vi "Autogenerated adjust limbus.vi"(0 "Range (Threshold 1)":cluster{"Lower value":sgl, "Upper value":sgl}={"Lower value"=140.0, "Upper value"=255.0}, 7 "error in":errorcluster) -> (20 "Fitted Circle (Find Circular Edge 1)":T2 {"Average SNR (dB)" format="%.2f"; "Average Strength" format="%.2f"; "Roundness (Real-World)" format="%.2f"; "Radius (Real-World)" format="%.2f"; "Center (Real-World)"."Y" format="%.2f"; "Center (Real-World)"."X" format="%.2f"; "Radius (Pixels)" format="%.2f"; "Center (Pixels)"."Y" format="%.2f"; "Center (Pixels)"."X" format="%.2f"}, 27 "error out":errorcluster)   [LabVIEW 2014]
uses:
  <vilib>/vision/Measure.llb/Edge Options.ctl
  <vilib>/vision/Measure.llb/Edge Polarity.ctl
  <vilib>/vision/NI_Vision_Development_Module.lvlib
panel:
  out "Image Out":T1(plugin-control)
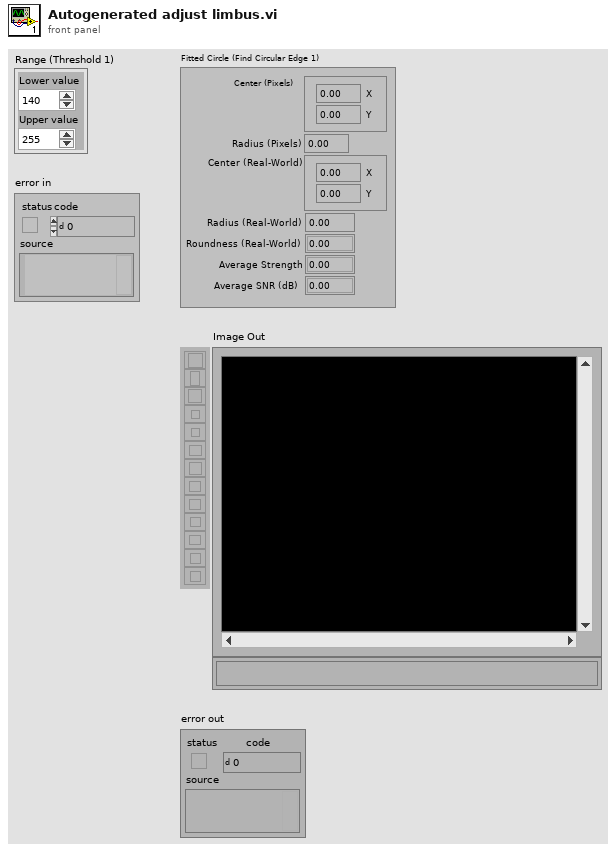
[diagram p1: front panel]
types:
  T1 = typedef "IMAQ Image.ctl" = refnum<image>
  T2 = cluster{"Center (Pixels)":cluster{"X":sgl, "Y":sgl}, "Radius (Pixels)":dbl, "Center (Real-World)":cluster{"X":sgl, "Y":sgl}, "Radius (Real-World)":dbl, "Roundness (Real-World)":dbl, "Average Strength":dbl, "Average SNR (dB)":dbl}
  T3 = typedef "Edge Options.ctl" = cluster{"Edge Polarity":T4, "Kernel Size":u32, "Width":u32, "Minimum Edge Strength":sgl, "Interpolation Type":enum32{"Zero Order", "Bilinear", "Quadratic", "Cubic", "Bilinear Fixed"}, "Data Processing Method":enum32{"Average", "Median"}}
  T4 = typedef "Edge Polarity.ctl" = u32
  T5 = cluster{"Search  Direction":u32, "Edge Options":T3, "Show Search Area":bool, "Show Search Lines":bool, "Show Edges Found":bool, "Show Result":bool, "Search Area Color":u32, "Search Lines Color":u32, "Edge Locations Color":u32, "Result Color":u32, "Overlay Group Name":string}
  T6 = cluster{"Process":enum16{"Get First Edge", "Get First + Last Edge", "Get All Edges", "Get Best Edge"}, "Step Size":i32, "Max Pixel Radius":i32}
  T7 = cluster{"Global Rectangle":i32[], "Contours":cluster{"ID":enum32{"External", "Internal"}, "Type":u32, "Coordinates":i32[]}[]}
  T8 = typedef "Image Type" = u32
  T9 = cluster{"histogram":u32[], "Minimal Value":sgl, "Maximal Value":sgl, "Starting Value":sgl, "Interval Width":sgl, "Mean Value":sgl, "Standard  Variation":sgl, "Area (pixels)":i32}
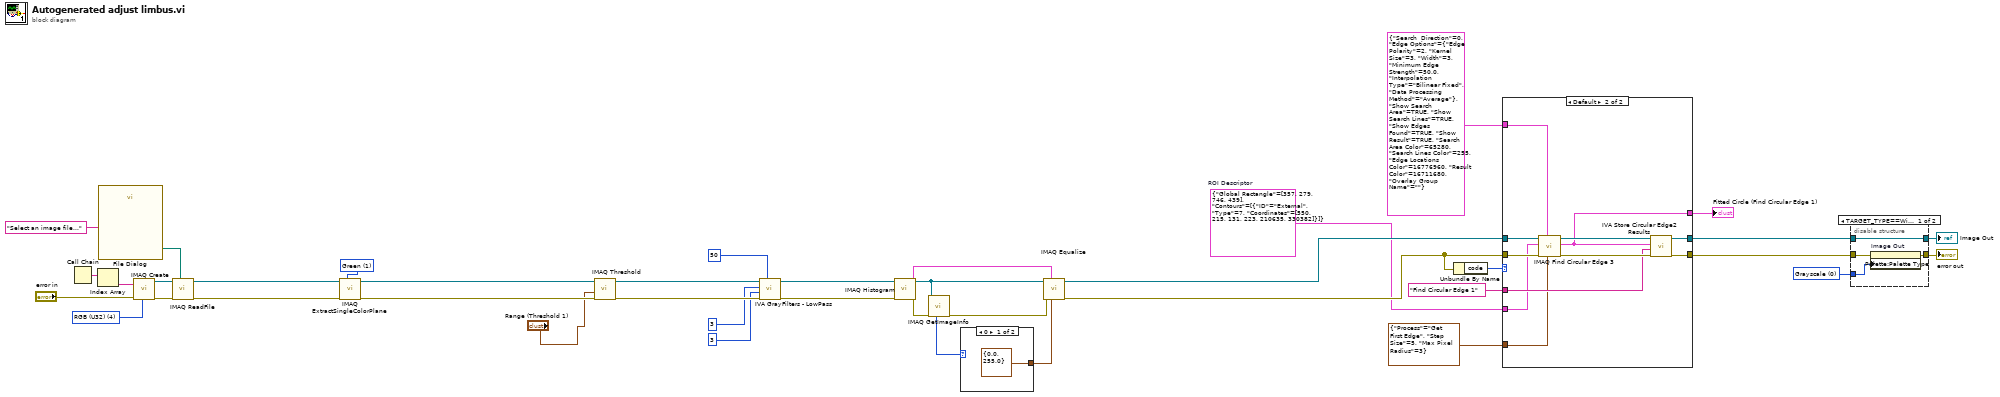
[diagram p0: block diagram]
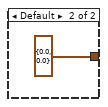
[diagram p4: hidden frame]
diagram:
  w1 = u32 0 items=["Grayscale", "Binary", "Gradient", "Rainbow", "Temperature", "User Defined"] ("Palette")
  w9 = T7 {"Global Rectangle"=[357, 279, 746, 439], "Contours"=[{"ID"=enum."External", "Type"=7, "Coordinates"=[550, 215, 131, 223, 210635, 330382]}]}  # ROI Descriptor
  w30 = 1 items=["Red", "Green", "Blue", "Hue", "Saturation", "Luminance", "Value", "Intensity"] ("Color Plane")
  w31 = T8 4 items=["Grayscale (U8)", "Grayscale (I16)", "Grayscale (SGL)", "Complex (CSG)", "RGB (U32)", "HSL (U32)", "RGB (U64)", "Grayscale (U16)"] ("Image Type")
  n1 = Call Chain() -> (call chain=w35:string[])
  n2 = Index Array(array=w35) -> (element=w34:string)  [unwired: 1 in]
  n3 = call "File Dialog"("prompt"="Select an image file...") -> ("selected path"=w32:path)  [unwired: 6 in, 8 out]
  n4 = call "IMAQ Create"("Image Name"=w34, "Image Type"=w31, "error in (no error)"="error in") -> ("New Image"=w38:T1, "error out"=w37:errorcluster)  [unwired: 1 in, 1 out]
  n5 = call "IMAQ ReadFile"("File Path"=w32, "error in (no error)"=w37, "Image"=w38) -> ("error out"=w39:errorcluster, "Image Out"=w29:T1)  [unwired: 2 in, 5 out]
  n6 = call "IMAQ ExtractSingleColorPlane"("Color Plane"=w30, "error in (no error)"=w39, "Image Src"=w29) -> ("error out"=w28:errorcluster, "Image Dst Out"=w26:T1)  [unwired: 1 in, 6 out]
  n7 = call "IMAQ Threshold"("error in (no error)"=w28, "Range"="Range (Threshold 1)", "Image Src"=w26) -> ("error out"=w25:errorcluster, "Image Dst Out"=w24:T1)  [unwired: 3 in, 4 out]
  n8 = call <vilib>:"IVA GrayFilters - LowPass.vi"("Tolerance"=50, "error in"=w25, "Filter size Y"=3, "Filter size X"=3, "Image In"=w24) -> ("error out"=w23:errorcluster, "Image Out"=w16:T1)  [unwired: 5 out]
  n9 = call "IMAQ Histogram"("error in (no error)"=w23, "Image"=w16) -> ("error out"=w15:errorcluster, "Histogram Report"=w18:T9)  [unwired: 3 in, 5 out]
  n10 = call "IMAQ GetImageInfo"("error in (no error)"=w15, "Image"=w16) -> ("error out"=w14:errorcluster, "Image Type"=w17:T8)  [unwired: 8 out]
  n11 = case shown="0" w17 {
    tunnel: [cluster{"Minimum":sgl, "Maximum":sgl} {"Minimum"=0.0, "Maximum"=255.0} ("Range") cluster{"Minimum":sgl, "Maximum":sgl} {"Minimum"=0.0, "Maximum"=0.0} ("Range")] -> w13
    frame 0 {
    }
    frame Default {
    }
  }
  n12 = call "IMAQ Equalize"("Range"=w13, "Histogram Report"=w18, "error in (no error)"=w14, "Image Src"=w16) -> ("error out"=w19:errorcluster, "Image Dst Out"=w12:T1)  [unwired: 2 in, 4 out]
  n13 = Unbundle By Name(w19) -> ("code"=w8:i32)
  n14 = case shown="Default" w8 {
    tunnel: T5 {"Search  Direction"=0, "Edge Options"={"Edge Polarity"=2, "Kernel Size"=3, "Width"=3, "Minimum Edge Strength"=50.0, "Interpolation Type"=enum."Bilinear Fixed", "Data Processing Method"=enum."Average"}, "Show Search Area"=TRUE, "Show Search Lines"=TRUE, "Show Edges Found"=TRUE, "Show Result"=TRUE, "Search Area Color"=65280, "Search Lines Color"=255, "Edge Locations Color"=16776960, "Result Color"=16711680, "Overlay Group Name"=""} ("Options") -> [_ w43]
    tunnel: w12 -> [w42 w53]
    tunnel: w19 -> [_ w52]
    tunnel: [_ w50] -> w11
    tunnel: [w42 w48] -> w3
    tunnel: "Find Circular Edge 1" ("Step Name") -> [_ w47]
    tunnel: w9 -> [_ w46]
    tunnel: T6 {"Process"=enum."Get First Edge", "Step Size"=5, "Max Pixel Radius"=3} ("Circle Fit Options") -> [_ w45]
    tunnel: [_ w44] -> w6
    frame -1074396199, -1074396198 {
      # "Discard Coordinate System Error"
    }
    frame Default {
      n15 = call "IMAQ Find Circular Edge 3"("Circle Fit Options"=w45, "Options"=w43, "error in (no error)"=w52, "ROI Descriptor"=w46, "Image"=w53) -> ("error out"=w51:errorcluster, "Fitted Circle"=w44:T2, "Image Out"=w49:T1)  [unwired: 2 in, 2 out]
      n16 = call <vilib>:"IVA Store Circular Edge2 Results.vi"("error in (no error)"=w51, "Step Name"=w47, "Fitted Circle"=w44, "Image in"=w49) -> ("error out"=w50:errorcluster, "Image dup"=w48:T1)  [unwired: 2 in, 4 out]
    }
  }
  "Fitted Circle (Find Circular Edge 1)" <- w6
  n17 = disable-structure "Conditional Disable Structure" shown="TARGET_TYPE==Windows" {
    disable-tunnel: w11 -> [w57 w58]
    disable-tunnel: [w56 w58] -> w4
    disable-tunnel: w3 -> [w55 w59]
    disable-tunnel: [w55 w59] -> w2
    disable-tunnel: w1 -> [w54 _]
    frame condition #0 (active) {
      n18 = property on="Image Out" class="ImageControl"(error in=w57, "Palette:Palette Type"=w54) -> (error out=w56:errorcluster)  [unwired: 1 in, 1 out]
    }
    frame condition #1 {
    }
  }
  "error out" <- w4
  "Image Out" <- w2
